vi "Lab3.vi"() -> ()   [LabVIEW 2011]
panel:
  out "XY Graph":cluster{dbl[], dbl[]}[](graph)
  in  "Xk":dbl
  in  "dx":dbl
  in  "X0":dbl
  in  "Ymin":dbl
  in  "Ymax":dbl
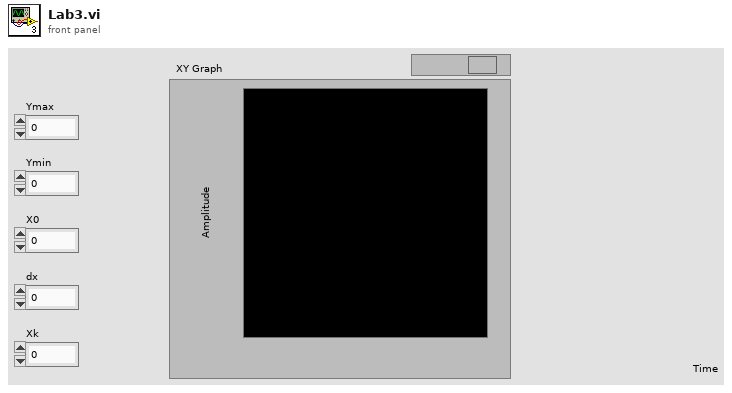
[diagram p1: front panel]
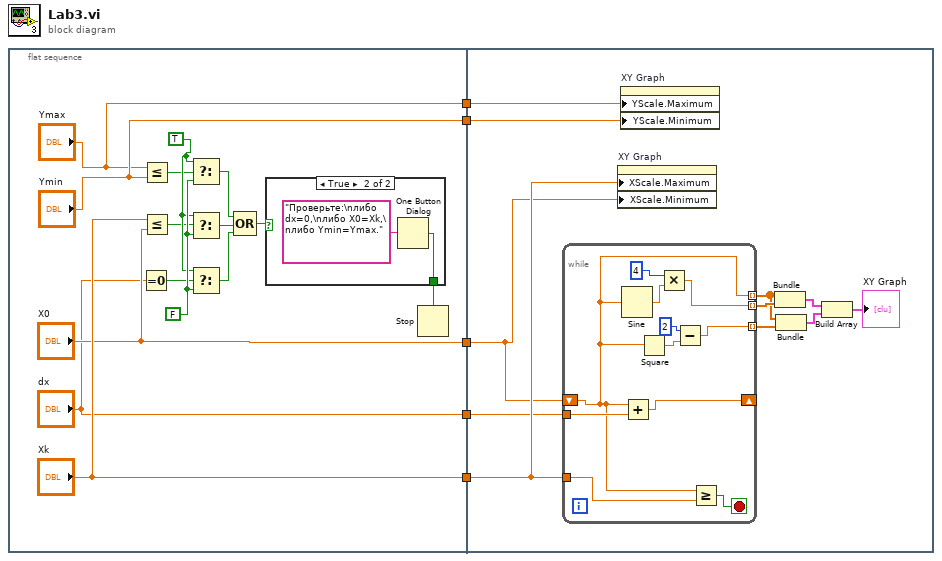
[diagram p0: block diagram]
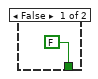
[diagram p2: hidden frame]
diagram:
  n1 = flat-sequence {
    tunnel: ["Ymin"] -> w5
    tunnel: ["Ymax"] -> w4
    tunnel: ["Xk"] -> w3
    tunnel: ["X0"] -> w2
    tunnel: ["dx"] -> w1
    tunnel: w5 -> [w31]
    tunnel: w4 -> [w30]
    tunnel: w3 -> [w29]
    tunnel: w2 -> [w28]
    tunnel: w1 -> [w27]
    frame #0 {
      w15 = FALSE
      w14 = TRUE
      n2 = Equal To 0?(x="dx") -> (x = 0?=w11:bool)
      n3 = Less Or Equal?(x="Ymax", y="Ymin") -> (x <= y?=w13:bool)
      n4 = Less Or Equal?(x="Xk", y="X0") -> (x <= y?=w12:bool)
      n5 = Select(t=w14, s=w13, f=w15) -> (s? t:f=w19:bool)
      n6 = Select(t=w14, s=w12, f=w15) -> (s? t:f=w18:bool)
      n7 = Select(t=w14, s=w11, f=w15) -> (s? t:f=w17:bool)
      n8 = Compound Arithmetic op=OR(w19, w18, w17) -> (w20:bool)
      n9 = case shown="True" w20 {
        tunnel: [FALSE w22] -> w16
        frame False {
        }
        frame True {
          n10 = One Button Dialog(message="Проверьте:\nлибо dx=0,\nлибо X0=Xk,\nлибо Ymin=Ymax.") -> (true=w22:bool)  [unwired: 1 in]
        }
      }
      n11 = Stop(stop? (T)=w16) -> ()
    }
    frame #1 {
      n12 = while {
        shift-right: [w42] -> _
        shift-left: w28 -> [w35]
        tunnel: w29 -> [w44]
        tunnel: w27 -> [w43]
        tunnel: [w35] -> w25 mode=indexing
        tunnel: [w39] -> w26 mode=indexing
        tunnel: [w36] -> w24 mode=indexing
        stop <- w45 stop-if-true
        n13 = Sine(x=w35) -> (sin(x)=w40:dbl)
        n14 = Add(x=w35, y=w43) -> (x+y=w42:dbl)
        n15 = Square(x=w35) -> (x^2=w37:dbl)
        n16 = Multiply(x=4, y=w40) -> (x*y=w39:dbl)
        n17 = Subtract(x=2, y=w37) -> (x-y=w36:dbl)
        n18 = Greater Or Equal?(x=w35, y=w44) -> (x >= y?=w45:bool)
      }
      n19 = property on="XY Graph" class="XYGraph (strict)"("XScale.Maximum"=w29, "XScale.Minimum"=w28) -> ()  [unwired: 2 in, 2 out]
      n20 = property on="XY Graph" class="XYGraph (strict)"("YScale.Maximum"=w30, "YScale.Minimum"=w31) -> ()  [unwired: 2 in, 2 out]
      n21 = Bundle(w25, w26) -> (w34:cluster{dbl[], dbl[]})  [unwired: 1 in]
      n22 = Bundle(w25, w24) -> (w33:cluster{dbl[], dbl[]})  [unwired: 1 in]
      n23 = Build Array(w34, w33) -> (→"XY Graph":cluster{dbl[], dbl[]}[])
    }
  }
